vi "colorFromRGB.vi"(6 "Blue":u8, 8 "error in (no error)":errorcluster, 9 "Green":u8, 10 "Red":u8, 11 "Color in":refnum<class "Color.lvclass">) -> (0 "error out":errorcluster, 2 "Color":u16, 3 "Color out":refnum<class "Color.lvclass">)   [LabVIEW 2020, in "RPI.SenseHat.Display.lvlib" / "Color.lvclass"]
doc: "Converts RGB color components to RGB565 color."
uses:
  Color.lvclass
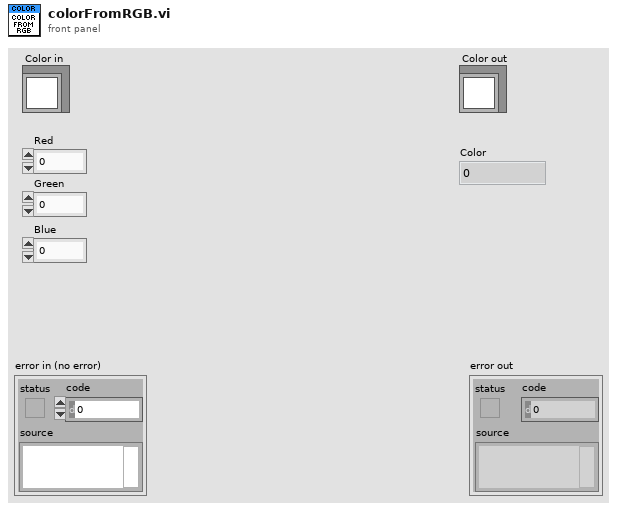
[diagram p1: front panel]
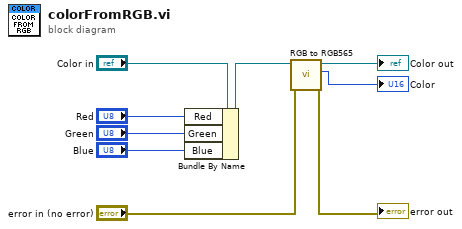
[diagram p0: block diagram]
diagram:
  n1 = Bundle By Name(cluster="Color in", "Red"="Red", "Green"="Green", "Blue"="Blue") -> (w5:refnum<class "Color.lvclass">)
  n2 = call "RGB to RGB565.vi"("error in (no error)"="error in (no error)", "Color in"=w5) -> ("error out"=→"error out":errorcluster, "Color"=→"Color":u16, "Color out"=→"Color out":refnum<class "Color.lvclass">)  [unwired: 7 in]
